vi "Update Points Done in Record.vi"(8 "Increment?":bool, 10 "Points Acquired":u16, 11 "Points to Acquire":u16) -> (0 "Points Done ?":bool, 2 "Points to Acquire > 0?":bool, 3 "Updated Points Acquired":u16)   [LabVIEW 2014]
panel:
  # "Copyright 2014 Vidrio Technologies\nScanImage 5 software is licensed under the Apache License, Version 2.0 (the \"License\"); you may not use any files contained\nwithin the ScanImage 5 release except in compliance with the License. You may obtain a copy of the License at\n http://www.apache.org/licenses/LICENSE-2.0\nUnless required by applicable law or agreed to in writing, software distributed under the License is distributed on an\n\"AS IS\" BASIS, WITHOUT WARRANTIES OR CONDITIONS OF ANY KIND, either express or implied. See the License for the\n specific language governing permissions and limitations under the License."
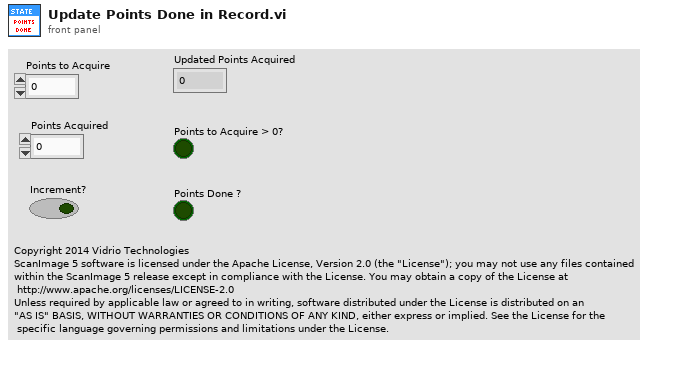
[diagram p1: front panel]
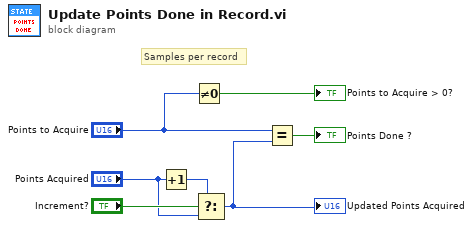
[diagram p0: block diagram]
diagram:
  # "Samples per record"
  n1 = Increment(x="Points Acquired") -> (x+1=w7:u16)
  n2 = Not Equal To 0?(x="Points to Acquire") -> (x != 0?=→"Points to Acquire > 0?":bool)
  n3 = Select(t=w7, s="Increment?", f="Points Acquired") -> (s? t:f=w4:u16)
  "Updated Points Acquired" <- w4
  n4 = Equal?(x="Points to Acquire", y=w4) -> (x = y?=→"Points Done ?":bool)
